vi "Challenge 1.vi"() -> ()   [LabVIEW 2019]
panel:
  out "Pressure Shunt":bool
  out "Vacuum Power":dbl
  out "HATCH Ejection Piston":bool
  in  "Eject HATCH":bool
  out "Timer (seconds)":dbl
  in  "Reset Timer":bool
  out "Intake Position":bool
  in  "Toggle Intake":bool
  out "Motor Power":dbl
  in  "Turn on Motor":bool
  # "Problem #1"
  # "Problem #2"
  # "Problem #3"
  # "Problem #4"
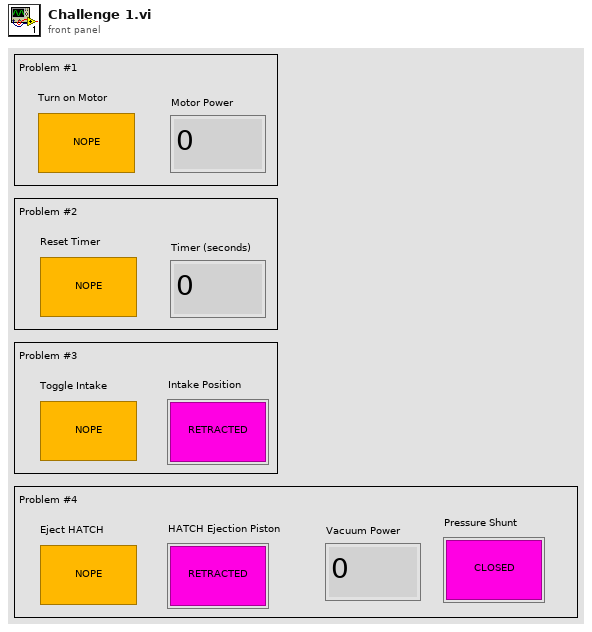
[diagram p1: front panel]
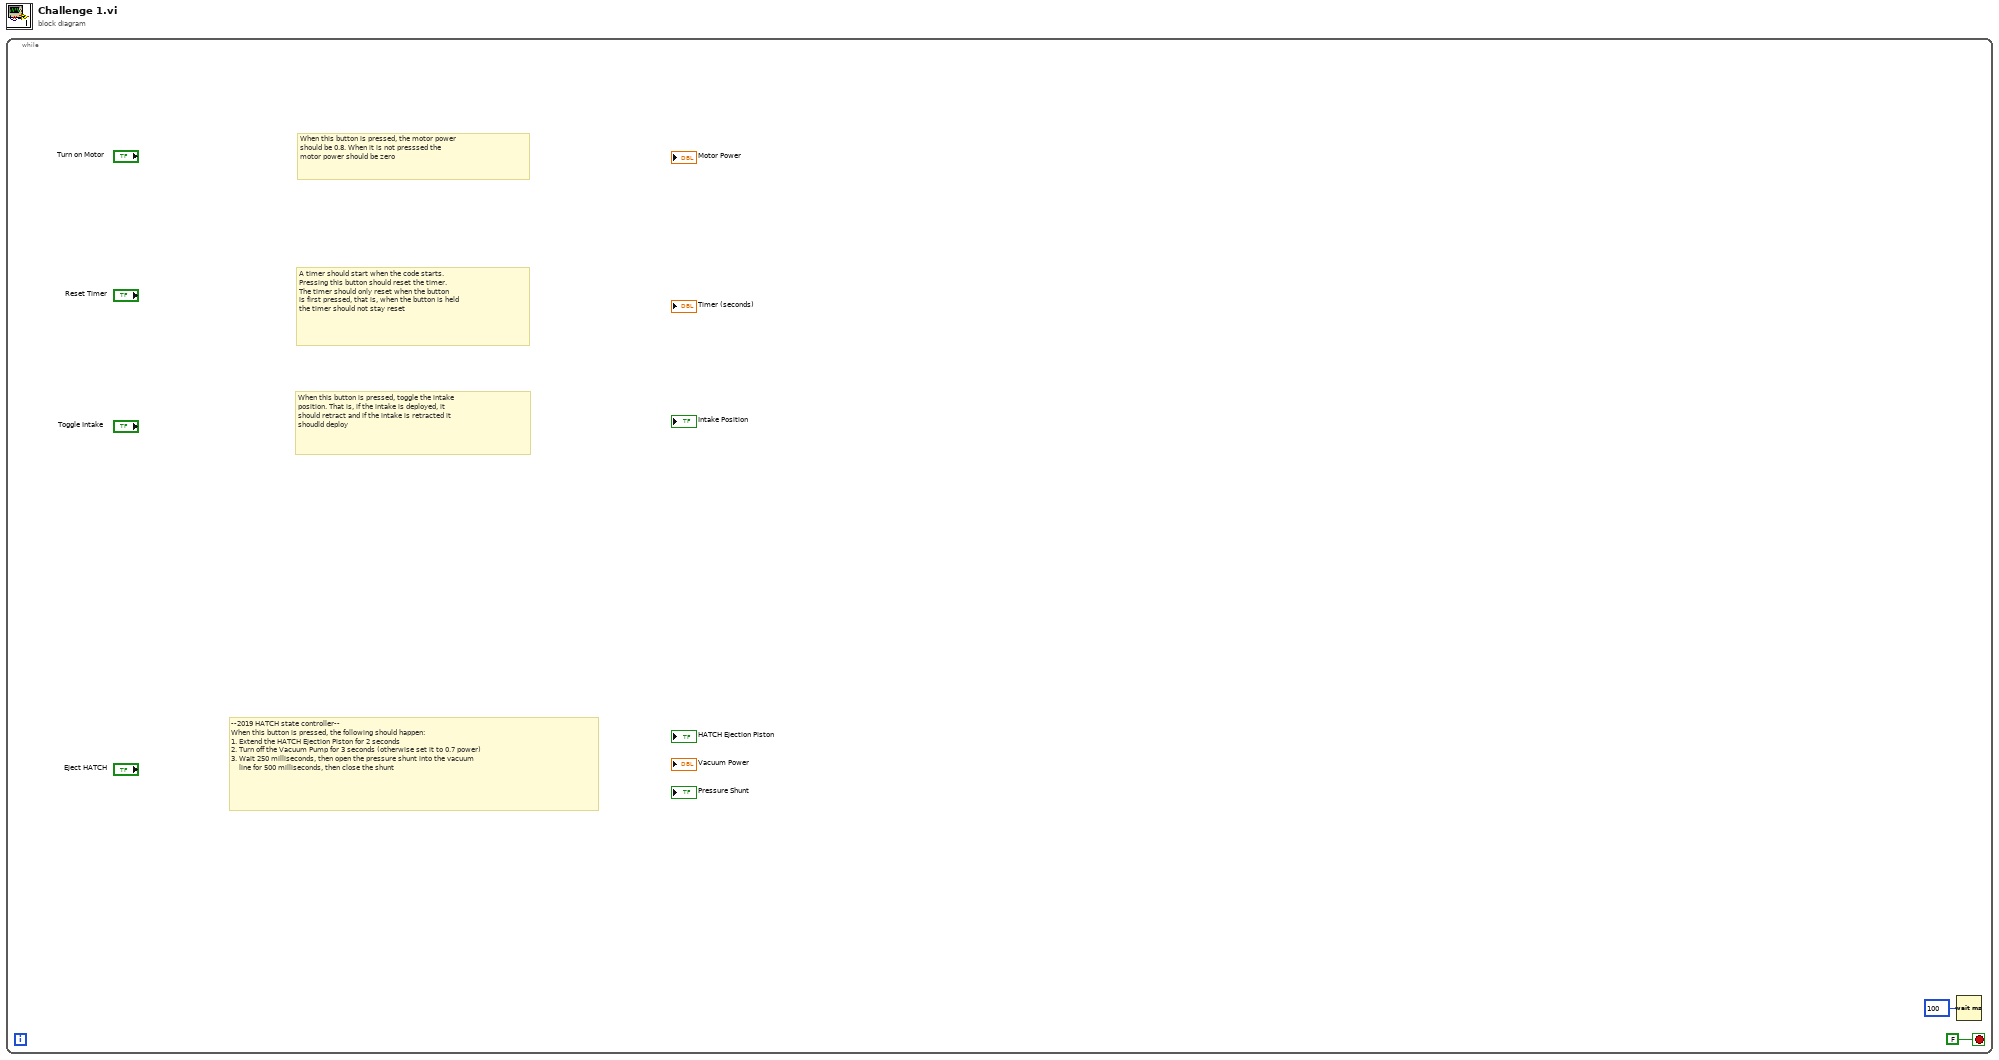
[diagram p0: block diagram]
diagram:
  n1 = while {
    stop <- FALSE stop-if-true
    # "--2019 HATCH state controller--\nWhen this button is pressed, the following should happen:\n1. Extend the HATCH Ejection Piston for 2 seconds\n2. Turn off the Vacuum Pump for 3 seconds (otherwise set it to 0.7 power)\n3. Wait 250 milliseconds, then open the pressure shunt into the vacuum\n    line for 500 milliseconds, then close the shunt"
    # "A timer should start when the code starts.\nPressing this button should reset the timer.\nThe timer should only reset when the button\nis first pressed, that is, when the button is held\nthe timer should not stay reset"
    # "When this button is pressed, toggle the intake \nposition. That is, if the intake is deployed, it \nshould retract and if the intake is retracted it\nshoudld deploy"
    # "When this button is pressed, the motor power\nshould be 0.8. When it is not presssed the \nmotor power should be zero"
    n2 = Wait (ms)(milliseconds to wait=u32 100) -> ()  [unwired: 1 out]
  }
